vi "Autonomous Independent.vi"   [LabVIEW 2018]
doc: "This VI is called when autonomous begins, and will automatically be terminated when autonomous ends. You can carry out timed or sensor driven robot movement independently without needing to return to the caller."
uses:
  Globals.vi
  <vilib>/Rock Robotics/Network Tables/NT Read String Array.vi
panel:
  # "Be sure to right-click and choose Data Operations>>Make Current Value default if you want to save the array values with the VI"
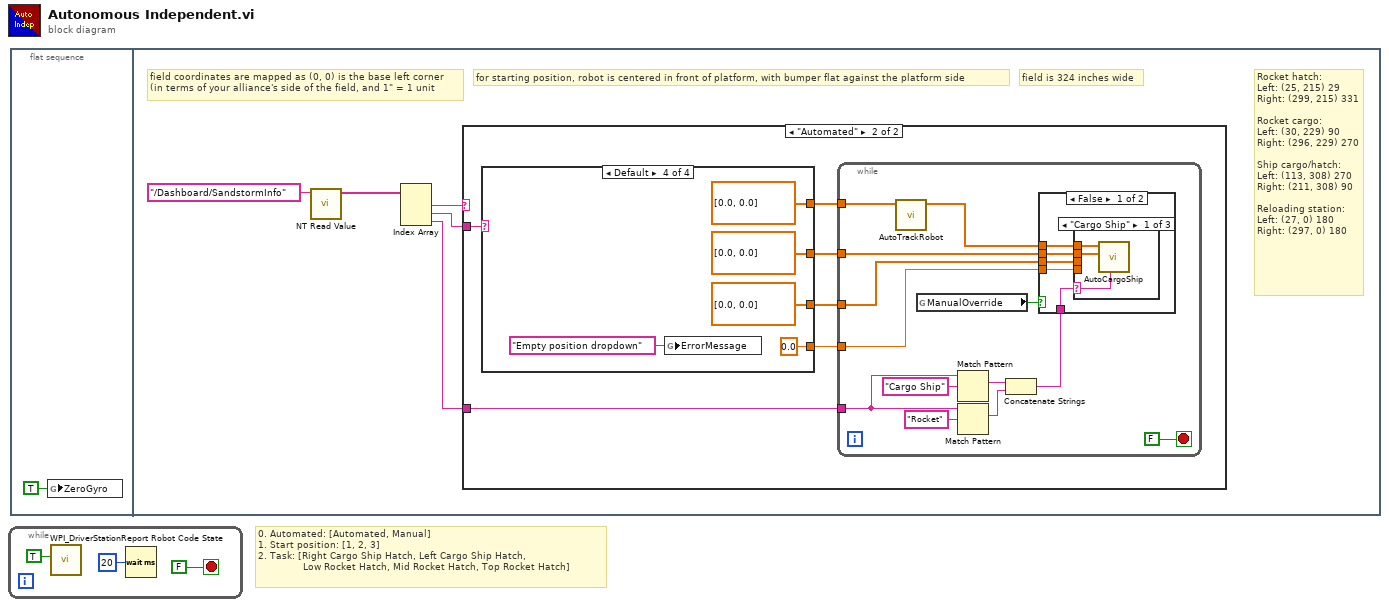
[diagram p0: block diagram]
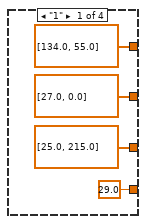
[diagram p3: hidden frame]
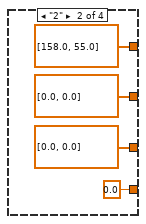
[diagram p4: hidden frame]
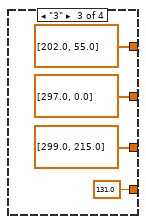
[diagram p5: hidden frame]
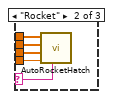
[diagram p6: hidden frame]
diagram:
  # "0. Automated: [Automated, Manual]\n1. Start position: [1, 2, 3]\n2. Task: [Right Cargo Ship Hatch, Left Cargo Ship Hatch,\n               Low Rocket Hatch, Mid Rocket Hatch, Top Rocket Hatch]"
  n1 = while {
    stop <- FALSE stop-if-true
    n2 = call <vilib>:"WPI_DriverStationReport Robot Code State.vi"("Autonomous"=TRUE) -> ()  [unwired: 10 in, 1 out]
    n3 = Wait (ms)(milliseconds to wait=u32 20) -> ()  [unwired: 1 out]
  }
  n4 = flat-sequence {
    frame #0 {
      n5 = global write "Globals.vi" "ZeroGyro"(TRUE ("ZeroGyro")) -> ()
    }
    frame #1 {
      # "Rocket hatch:\nLeft: (25, 215) 29\nRight: (299, 215) 331\n\nRocket cargo:\nLeft: (30, 229) 90\nRight: (296, 229) 270\n\nShip cargo/hatch:\nLeft: (113, 308) 270\nRight: (211, 308) 90\n\nReloading station:\nLeft: (27, 0) 180\nRight: (297, 0) 180"
      # "field is 324 inches wide"
      # "for starting position, robot is centered in front of platform, with bumper flat against the platform side"
      # "field coordinates are mapped as (0, 0) is the base left corner\n(in terms of your alliance's side of the field, and 1\" = 1 unit"
      n6 = call-poly <vilib>:"NT Read Value.vi"("Name"="/Dashboard/SandstormInfo") -> ("String Array"=w8:string[])  [unwired: 9 in, 1 out]
      n7 = Index Array(array=w8) -> (element #1=w6:string, element #2=w7:string, element #3=w5:string)  [unwired: 3 in]
      n8 = case shown="\"Automated\"" w6 {
        tunnel: w7 -> [_ w14]
        tunnel: w5 -> [_ w13]
        frame "Manual", Default {
        }
        frame "Automated" {
          n9 = case shown="Default" w14 {
            tunnel: [dbl[] [134.0, 55.0] dbl[] [158.0, 55.0] dbl[] [202.0, 55.0] dbl[] [0.0, 0.0]] -> w15
            tunnel: [dbl[] [27.0, 0.0] dbl[] [0.0, 0.0] dbl[] [297.0, 0.0] dbl[] [0.0, 0.0]] -> w12
            tunnel: [dbl[] [25.0, 215.0] dbl[] [0.0, 0.0] dbl[] [299.0, 215.0] dbl[] [0.0, 0.0]] -> w11
            tunnel: [29.0 0.0 131.0 0.0] -> w10
            frame "1" {
            }
            frame "2" {
            }
            frame "3" {
            }
            frame Default {
              n10 = global write "Globals.vi" "ErrorMessage"("Empty position dropdown" ("ErrorMessage")) -> ()
            }
          }
          n11 = while {
            tunnel: w15 -> [w37]
            tunnel: w13 -> [w40]
            tunnel: w12 -> [w43]
            tunnel: w11 -> [w35]
            tunnel: w10 -> [w34]
            stop <- FALSE stop-if-true
            n12 = call "AutoTrackRobot.vi"("StartCoordinates"=w37) -> ("Coordinates"=w45:dbl[])  [unwired: 10 in]
            n13 = global read "Globals.vi" "ManualOverride"() -> (w44:bool)
            n14 = Match Pattern(string=w40, regular expression="Cargo Ship") -> (match substring=w39:string)  [unwired: 1 in, 3 out]
            n15 = Match Pattern(string=w40, regular expression="Rocket") -> (match substring=w38:string)  [unwired: 1 in, 3 out]
            n16 = Concatenate Strings(w39, w38) -> (w36:string)
            n17 = case shown="False" w44 {
              tunnel: w45 -> [w49 _]
              tunnel: w43 -> [w50 _]
              tunnel: w36 -> [w48 _]
              tunnel: w35 -> [w47 _]
              tunnel: w34 -> [w46 _]
              frame False {
                n18 = case shown="\"Cargo Ship\"" w48 {
                  selector: w48 -> [w51 w58 _]
                  tunnel: w50 -> [w52 w55 _]
                  tunnel: w49 -> [w53 w54 _]
                  tunnel: w47 -> [_ w56 _]
                  tunnel: w46 -> [_ w57 _]
                  frame "Cargo Ship" {
                    n19 = call "AutoCargoShip.vi"("DestinationName"=w51, "FeederStation"=w52, "Coordinates"=w53) -> ()  [unwired: 9 in]
                  }
                  frame "Rocket" {
                    n20 = call "AutoRocketHatch.vi"("DestinationName"=w58, "DestinationAngle"=w57, "DestinationPort"=w56, "FeederStation"=w55, "Coordinates"=w54) -> ()  [unwired: 7 in]
                  }
                  frame "", Default {
                  }
                }
              }
              frame True {
              }
            }
          }
        }
      }
    }
  }
